vi "MJ_Fun.vi"(9 "Views":T2 {"mag/phase" items=["FRF", "rad phase unwrapped", "deg phase unwrapped", "rad phase wrapped", "deg phase wrapped", "White Plots", "MJ Map", "Real and Imaginary"]; "Bands" items=["No Bands", "", "Test2", "test3", "Test"]; "Smoothing" items=["No smoothing"=0, "1/4 semitone"=25, "1/2 semitone"=50, "1 semitone"=100, "2 semitones"=200, "Woodhouse"=19]; "View Type" items=["As measured", "Normalize", "Separate", "Complex Average", "Real Average", "Standard Deviation"]}, 10 "Old Files":T4[](array[typedef])) -> ()   [LabVIEW 2022 SP3]
uses:
  Curtin1_Label.ctl
  <vilib>/Math Plots/2D Math Plots/2D Compass/2D Compass XCtrl/2D Compass.xctl
  GraphType.ctl
  <vilib>/Math Plots/2D Math Plots/2D Compass/2D Compass Datatype/Public/Plot Helper (Vector).vi
  <vilib>/Math Plots/2D Math Plots/2D Compass/2D Compass Datatype/2D Compass Datatype.lvclass
panel:
  in  "frequency":u32(slide) scale=200.0..10000.0
  in  "# positions":u32=12
  out "2D Compass":refnum<class "2D Plot Datatype.lvclass">[](xcontrol)
  out "r":dbl[](array[numeric])
  in  "Color Table":T3(ring)=enum."Rainbow"
  in  "Data Set":u16(ring) items=["Betts Strad H_002.trf", "Betts Strad H_002.trf", "Betts Strad H_003.trf", "Betts Strad H_003.trf", "Betts Strad H_004.trf", "Betts Strad H_004.trf", "Betts Strad H_005.trf", "Betts Strad H_005.trf", "Betts Strad H_006.trf"]
  out "2D plot":dbl[][](graph)
  # "Welcome to MJ's Plot\n\nThis is a plot with each row being a different run number (as ordered in the data set listing below).  The radial plot lets you look at the magnidtude of any frequency as a function of angle (assuming you chose different positions for each of your data sets - default is 12 positions)."
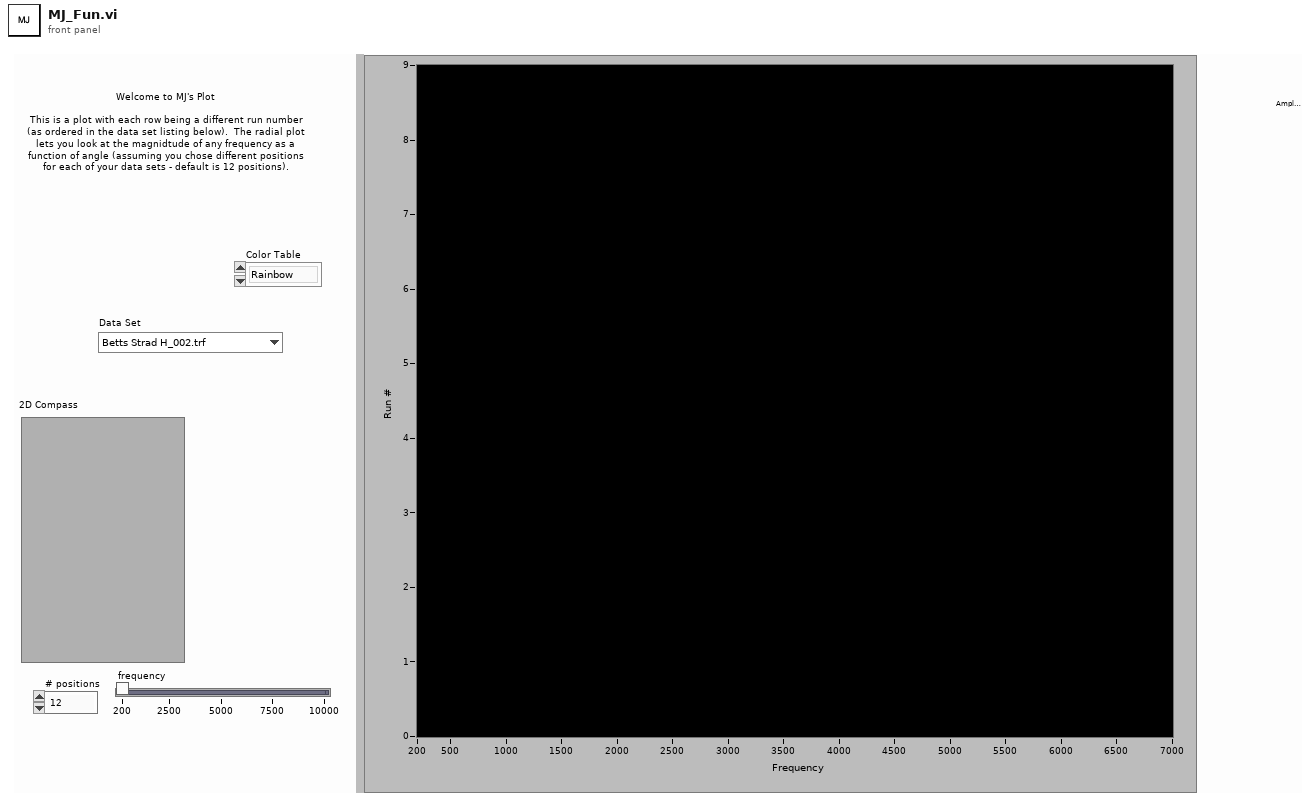
[diagram p1: front panel]
types:
  T1 = typedef "GraphType.ctl" = u16
  T2 = cluster{"View Type":u16, "Smoothing":u16, "Bands":u16, "New Band":bool, "rescale Y":bool, "rescale X":bool, "X_Low":dbl, "X_High":dbl, "dB Range":dbl, "Excel":bool, "Y Scaling":bool, "X Scaling":bool, "mag/phase":T1}
  T3 = enum16{"Apricot", "Carnation", "Ether", "Greyscale", "Greyscale-banded", "Hot Metal", "Lava Waves", "Mac", "Morning Glory", "Rainbow", "Rainbow-banded", "Rainbow-inverted", "Rainbow-striped", "Saturn", "Seismic", "Space"}
  T4 = typedef "Curtin1_Label.ctl" = cluster{"Show?":bool, "Name":string, "Color":u32, "Path":path, "Show Notes":bool}
  T5 = cluster{"Start freq":dbl, "Hz resolution":dbl, cdb[]}
  T6 = cluster{dbl, "df":dbl, "Power Spectrum (V^2 rms)":dbl[]}[]
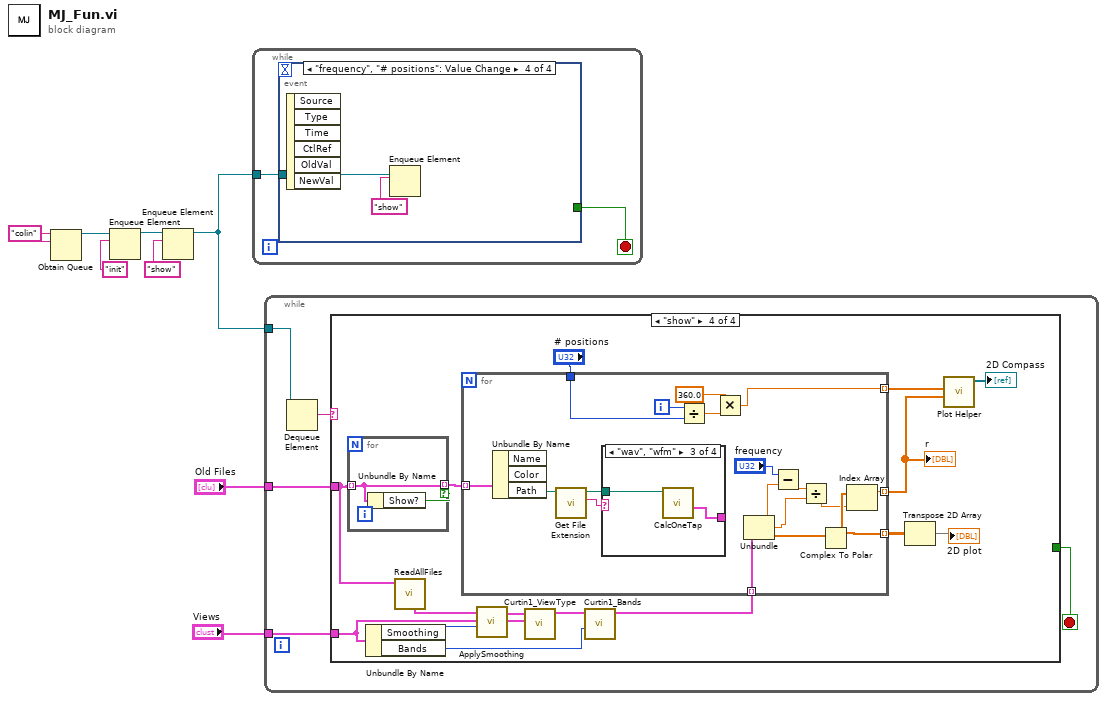
[diagram p0: block diagram]
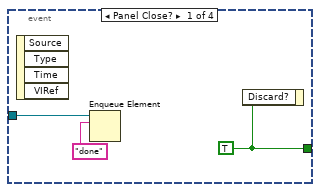
[diagram p2: hidden frame]
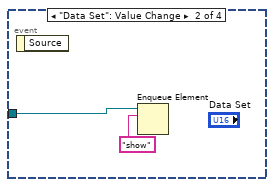
[diagram p3: hidden frame]
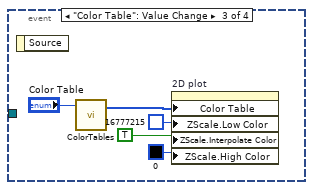
[diagram p4: hidden frame]
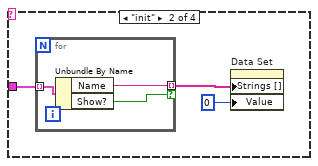
[diagram p6: hidden frame]
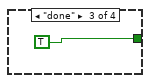
[diagram p7: hidden frame]
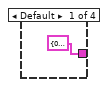
[diagram p8: hidden frame]
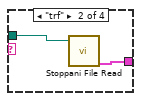
[diagram p9: hidden frame]
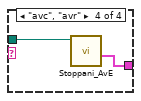
[diagram p10: hidden frame]
diagram:
  w8 = "colin" ("name (unnamed)")
  n1 = Obtain Queue(name (unnamed)=w8, element data type=w8) -> (queue out=w3:refnum<queue>)  [unwired: 3 in, 2 out]
  n2 = Enqueue Element(queue=w3, element="init") -> (queue out=w2:refnum<queue>)  [unwired: 2 in, 2 out]
  n3 = Enqueue Element(queue=w2, element="show") -> (queue out=w6:refnum<queue>)  [unwired: 2 in, 2 out]
  n4 = while {
    tunnel: w6 -> [w9]
    stop <- w10 stop-if-true
    n5 = event shown="[3] \"frequency\", \"# positions\": Value Change" {
      selector: _ -> [_ _ _ _]
      dyn-events: _ -> [_ _ _ _]
      timeout: _ -> [_ _ _ _]
      tunnel: [w11 _ _ _] -> w10
      tunnel: w9 -> [w12 w14 _ w21]
      event Panel Close? {
        w11 = TRUE
        n6 = event-data() -> ()  [unwired: 1 in, 4 out]
        n7 = Enqueue Element(queue=w12, element="done") -> ()  [unwired: 2 in, 3 out]
        n8 = event-data("Discard?"=w11) -> ()  [unwired: 1 in, 1 out]
      }
      event "Data Set": Value Change {
        n9 = event-data() -> ()  [unwired: 1 in, 1 out]
        n10 = Enqueue Element(queue=w14, element="show") -> ()  [unwired: 2 in, 3 out]
      }
      event "Color Table": Value Change {
        n11 = event-data() -> ()  [unwired: 1 in, 1 out]
        n12 = call "ColorTables.vi"("Color Table"="Color Table") -> ("Color Table Out"=w20:u32[])  [unwired: 2 in]
        n13 = property on="2D plot" class="IntGraph (strict)"("Color Table"=w20, "ZScale.Low Color"=u32 16777215 ("Z Scale.Low Color"), "ZScale.Interpolate Color"=TRUE ("Z Scale.Interpolate Color"), "ZScale.High Color"=u32 0 ("Z Scale.High Color")) -> ()  [unwired: 2 in, 2 out]
      }
      event "frequency", "# positions": Value Change {
        n14 = event-data() -> ()  [unwired: 1 in, 6 out]
        n15 = Enqueue Element(queue=w21, element="show") -> ()  [unwired: 2 in, 3 out]
      }
    }
  }
  n16 = while {
    tunnel: w6 -> [w27]
    tunnel: "Old Files" -> [w24]
    tunnel: "Views" -> [w23]
    stop <- w25 stop-if-true
    n17 = Dequeue Element(queue=w27) -> (element=w26:string)  [unwired: 2 in, 3 out]
    n18 = case shown="\"show\"" w26 {
      tunnel: [_ _ TRUE _] -> w25
      tunnel: w24 -> [_ w30 _ w39]
      tunnel: w23 -> [_ _ _ w37]
      frame Default {
      }
      frame "init" {
        n19 = for {
          tunnel: w30 -> [w33] mode=indexing
          tunnel: [w32] -> w29 mode=indexing if=w31
          n20 = Unbundle By Name(w33) -> ("Name"=w32:string, "Show?"=w31:bool)
        }
        n21 = property on="Data Set" class="Ring (strict)"("Strings []"=w29, "Value"=0) -> ()  [unwired: 2 in, 2 out]
      }
      frame "done" {
      }
      frame "show" {
        n22 = for {
          tunnel: w39 -> [w50] mode=indexing
          tunnel: [w50] -> w49 mode=indexing if=w51
          n23 = Unbundle By Name(w50) -> ("Show?"=w51:bool)
        }
        n24 = Unbundle By Name(w37) -> ("Smoothing"=w38:u16, "Bands"=w36:u16)
        n25 = call "ReadAllFiles.vi"("Files"=w39) -> ("data"=w42:cluster{"t0":dbl, "df":dbl, "Y":cdb[]}[])  [unwired: 5 in, 5 out]
        n26 = call "ApplySmoothing.vi"("Smoothing"=w38, "Complex FRF"=w42) -> ("Complex FRF Out"=w41:cluster{dbl, "df":dbl, cdb[]}[])  [unwired: 9 in]
        n27 = call "Curtin1_ViewType.vi"("Settings"=w37, "FRF in"=w41) -> ("FRF Out"=w40:cluster{dbl, "df":dbl, dbl[]}[])  [unwired: 8 in, 1 out]
        n28 = call "Curtin1_Bands.vi"("Bands"=w36, "Magnitude"=w40) -> ("Filter"=w35:T6)  [unwired: 8 in, 1 out]
        n29 = for {
          tunnel: w49 -> [w65] mode=indexing
          tunnel: [w56] -> w48 mode=indexing
          tunnel: "# positions" -> [w53]
          tunnel: [w61] -> w44 mode=indexing
          tunnel: [w55] -> w43 mode=indexing
          tunnel: w35 -> [w52] mode=indexing
          i -> [w64]
          n30 = Unbundle By Name(w65) -> ("Path"=w69:path)  [unwired: 2 out]
          n31 = call <vilib>:"Get File Extension.vi"("file"=w69) -> ("lowercase file extension"=w67:string, "dup file"=w68:path)  [unwired: 6 in, 3 out]
          n32 = case shown="\"wav\", \"wfm\"" w67 {
            tunnel: [T5 {"Start freq"=0.0, "Hz resolution"=0.0, []} ("Waveform Graph") w71 w73 w76] -> _
            tunnel: w68 -> [_ w72 w74 w75]
            frame Default {
            }
            frame "trf" {
              n33 = call "Stoppani File Read.vi"("String in"=w72) -> ("Complex FRF"=w71:cluster{"t0":dbl, "dt":dbl, "Y":cdb[]})  [unwired: 2 in, 3 out]
            }
            frame "wav", "wfm" {
              n34 = call "CalcOneTap.vi"("wavform file"=w74) -> ("Complex FRF"=w73:cluster{dbl, "df":dbl, cdb[]})  [unwired: 7 in, 3 out]
            }
            frame "avc", "avr" {
              n35 = call "Stoppani_AvE.vi"("file (use dialog)"=w75) -> ("Complex FRF"=w76:cluster{"t0":dbl, "df":dbl, "Y":cdb[]})  [unwired: 7 in, 3 out]
            }
          }
          n36 = Divide(x=w64, y=w53) -> (x/y=w63:dbl)
          n37 = Multiply(x=360.0, y=w63) -> (x*y=w61:dbl)
          n38 = Unbundle(w52) -> (w59:dbl, "df"=w57:dbl, "Power Spectrum (V^2 rms)"=w66:dbl[])
          n39 = Subtract(x="frequency", y=w59) -> (x-y=w58:dbl)
          n40 = Divide(x=w58, y=w57) -> (x/y=w54:dbl)
          n41 = Complex To Polar(r * e^(i*theta)=w66) -> (r=w56:dbl[])  [unwired: 1 out]
          n42 = Index Array(array=w56, index=w54) -> (element=w55:dbl)
        }
        "r" <- w43
        n43 = Transpose 2D Array(2D array=w48) -> (transposed array=→"2D plot":dbl[][])
        n44 = call-poly <vilib>:"Plot Helper.vi"("radius vector"=w43, "theta vector"=w44) -> ("2D Plot Class Obj Array out"=→"2D Compass":refnum<class "2D Plot Datatype.lvclass">[])  [unwired: 2 in, 7 out]
      }
    }
  }
